vi "CS_cRIO-PB_DP-Master_ModuleProperties.vi"(0 "FPGA VI Reference":T2, 11 "Error":errorcluster) -> (4 "FPGA VI Reference out":T2, 8 "cRIO-PB Module":T1 {"ModuleID" format="%.0x"; "VendorID" format="%.0x"}, 15 "Error out":errorcluster)   [LabVIEW 2013, in "dynamic profibus.lvlib"]
uses:
  dynamic profibus.lvlib
  <vilib>/rvi/interface/nirviReadWriteControl/nirviReadWriteControl.xnode
  fpga reference.ctl
  <vilib>/rvi/errors/niLvFpgaAdjustHostInterfaceError.vi
  <vilib>/rvi/interface/Simulation/niFpgaSimulationCallBeginRW.vi
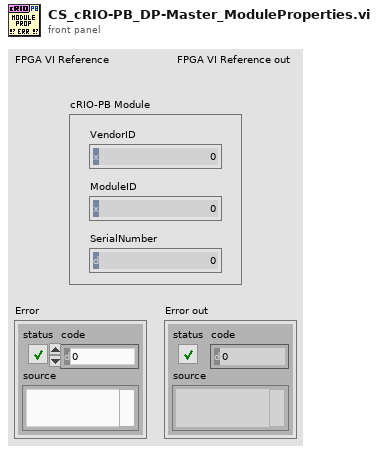
[diagram p1: front panel]
types:
  T1 = cluster{"VendorID":u16, "ModuleID":u16, "SerialNumber":u32}
  T2 = typedef "dynamic profibus.lvlib/fpga reference.ctl" = refnum<k20>
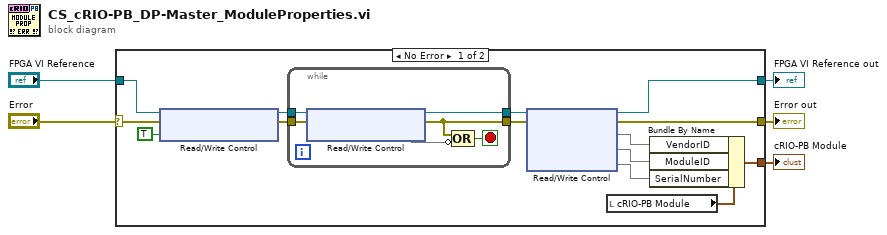
[diagram p0: block diagram]
diagram:
  n1 = case shown="No Error" "Error" {
    selector: "Error" -> [w16 w26]
    tunnel: "FPGA VI Reference" -> [w17 w27]
    tunnel: [w10 w27] -> w3
    tunnel: [w9 w26] -> w2
    tunnel: [w18 _] -> w1
    frame No Error {
      n2 = xnode "Read/Write Control"("FPGA VI Reference In"=w17, "error in"=w16, "cRIO-PB Properties"=TRUE ("GetData")) -> ("FPGA VI Reference Out"=w14:T2, "error out"=w15:errorcluster)
      n3 = while {
        tunnel: w15 -> [w24]
        tunnel: w14 -> [w23]
        tunnel: [w21] -> w11
        tunnel: [w22] -> w12
        stop <- w25 stop-if-true
        n4 = xnode "Read/Write Control"("FPGA VI Reference In"=w23, "error in"=w24) -> ("FPGA VI Reference Out"=w22:T2, "error out"=w21:errorcluster, "cRIO-PB Properties"=w20)
        n5 = Compound Arithmetic op=OR(w21, invert w20) -> (w25:bool)
      }
      n6 = xnode "Read/Write Control"("FPGA VI Reference In"=w12, "error in"=w11) -> ("FPGA VI Reference Out"=w10:T2, "error out"=w9:errorcluster, "VendorID"=w7, "ModuleID"=w6, "SerialNumber"=w8)
      n7 = local read "cRIO-PB Module"() -> (w19:T1)
      n8 = Bundle By Name(cluster=w19, "VendorID"=w7, "ModuleID"=w6, "SerialNumber"=w8) -> (w18:T1)
    }
    frame Error {
    }
  }
  "FPGA VI Reference out" <- w3
  "Error out" <- w2
  "cRIO-PB Module" <- w1
